vi "Test.vi"   [LabVIEW 2015]
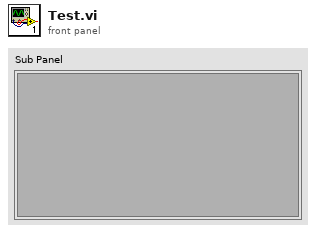
[diagram p1: front panel]
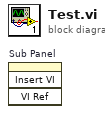
[diagram p0: block diagram]
diagram:
  n1 = invoke on="Sub Panel" class="SubPanel" method="Insert VI"() -> ()  [unwired: 4 in, 4 out]
